vi "Trigger Instr View.vi"(8 "error in":errorcluster, 9 "New Value":u16, 10 "Old Value":u16, 11 "Instruments in":refnum<class "Instruments.lvclass">) -> (0 "error out":errorcluster, 3 "Instruments out":refnum<class "Instruments.lvclass">)   [LabVIEW 2023, in "Instruments.lvlib" / "Instruments.lvclass"]
uses:
  Library/Instruments.lvclass
  Library/Instruments.lvclass/Instruments.ctl
  builds/Engine/Engine.lvlibp/Project/Engine.lvclass
  C:/Users/Public/Documents/Development/builds/Engine/Engine.lvlibp/Project/Engine.lvclass
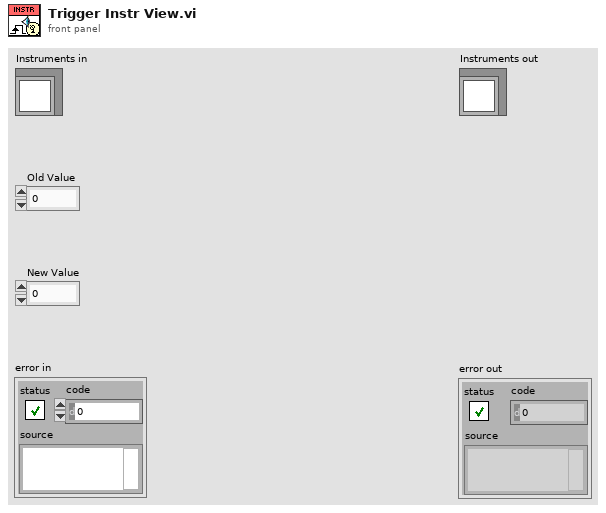
[diagram p1: front panel]
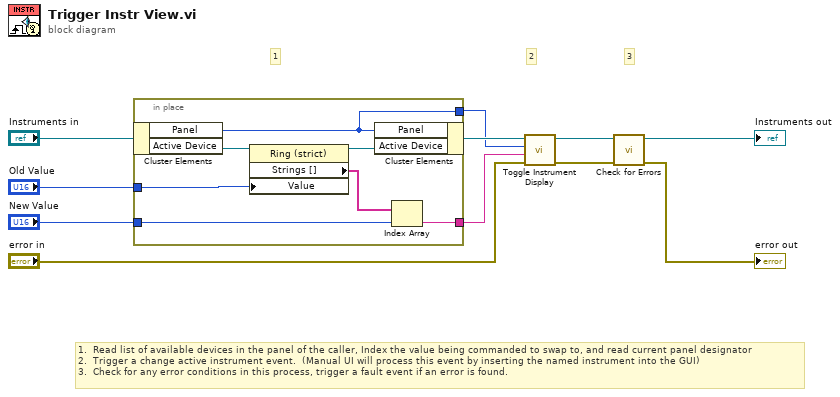
[diagram p0: block diagram]
diagram:
  # "1.  Read list of available devices in the panel of the caller, Index the value being commanded to swap to, and read current panel designator\n2.  Trigger a change active instrument event.  (Manual UI will process this event by inserting the named instrument into the GUI)\n3.  Check for any error conditions in this process, trigger a fault event if an error is found."
  # "3"
  # "2"
  # "1"
  n1 = in-place {
    in-place-border: "Old Value" -> [w16]
    in-place-border: "New Value" -> [w14]
    in-place-border: [w13] -> w7
    in-place-border: [w12] -> w6
    n2 = in-place-cluster #1("Instruments in") -> ("Panel"=w12:i32, "Active Device"=w18:refnum<vi>)
    n3 = property class="Ring (strict)"(reference=w18, "Value"=w16) -> (reference out=w17:refnum<vi>, "Strings []"=w15:string[])  [unwired: 1 in, 1 out]
    n4 = in-place-cluster #1("Panel"=w12, "Active Device"=w17) -> (w8:refnum<class "Instruments.lvclass">)
    n5 = Index Array(array=w15, index=w14) -> (element=w13:string)
  }
  n6 = call "Toggle Instrument Display.vi"("error in"="error in", "Identifier"=w7, "Panel"=w6, "Engine in"=w8) -> ("error out"=w3:errorcluster, "Engine out"=w4:refnum<class "Instruments.lvclass">)  [unwired: 6 in]
  n7 = call "Check for Errors.vi"("error in"=w3, "Engine in"=w4) -> ("error out"=→"error out":errorcluster, "Engine out"=→"Instruments out":refnum<class "Instruments.lvclass">)  [unwired: 8 in]
